vi "InitializeSteering.vi"(8 "error in (no error)":errorcluster, 10 "Steering PID Gains":T1={"proportional gain (Kc)"=100.0, "integral time (Ti, min)"=0.0, "derivative time (Td, min)"=37.0}, 11 "Encoder Initial Position":dbl) -> (0 "error out":errorcluster)   [LabVIEW 2014]
uses:
  <vilib>/Rock Robotics/WPI/CAN/TalonSRX/WPI_CANTalonSRX_APIControlMode.ctl
  <vilib>/Rock Robotics/WPI/CAN/TalonSRX/WPI_CANTalonSRX_APIFeedbackSelect.ctl
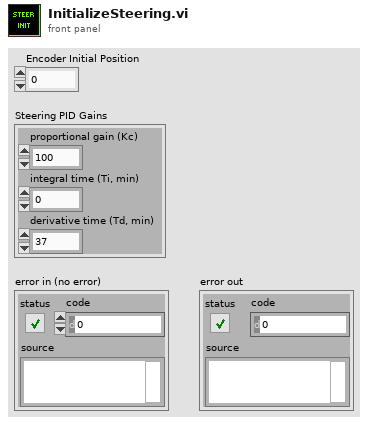
[diagram p1: front panel]
types:
  T1 = cluster{"proportional gain (Kc)":dbl, "integral time (Ti, min)":dbl, "derivative time (Td, min)":dbl}
  T2 = typedef "WPI_CANTalonSRX_APIFeedbackSelect.ctl" = enum16{"Digital Quadrature Encoder", "Analog Potentiometer", "Analog Encoder"}
  T3 = typedef "WPI_CANTalonSRX_APIControlMode.ctl" = enum8{"Percent VBus", "Speed", "Position", "Slave", "Unchanged / Invalid"}
  T4 = typedef "WPI_SwitchDevRef.ctl" = cluster{"DevStatus":errorcluster, "DIO Channel":T5, "Controller":T6, "CntIndex":T7, "Normally Closed":bool}
  T5 = typedef "FPGA_DIOChannel.ctl" = enum8{"DIO 0", "DIO 1", "DIO 2", "DIO 3", "DIO 4", "DIO 5", "DIO 6", "DIO 7", "DIO 8", "DIO 9", "DIO MXP 0", "DIO MXP 1", "DIO MXP 2", "DIO MXP 3", "DIO MXP 4", "DIO MXP 5", "DIO MXP 6", "DIO MXP 7", "DIO MXP 8", "DIO MXP 9", "DIO MXP 10", "DIO MXP 11", "DIO MXP 12", "DIO MXP 13", "DIO MXP 14", "DIO MXP 15", "Invalid"}
  T6 = typedef "FPGA_TypedefDigitalModule.ctl" = enum16{"Controller 1"}
  T7 = typedef "FPGA_CounterCtrSystemIndex.ctl" = enum8{"Ctr 0", "Ctr 1", "Ctr 2", "Ctr 3", "Ctr 4", "Ctr 5", "Ctr 6", "Ctr 7", "Invalid"}
  T8 = typedef "WPI_MotorControlDeviceRef.ctl" = cluster{"DeviceStatus":errorcluster, "Type":T9, "PWM":cluster{"Controller":T6, "PWM Channel":T10, "DeadBand":T11}, "CAN":cluster{"Device Number":u8, "Control Mode":T12, "Semaphore":T13, "Max Vout":dbl, "TalonSRX Control Mode":T3}, "Invert":bool, "TransformRef":T14, "InvTransformRef":T14}
  T9 = typedef "WPI_MotorControlType.ctl" = enum16{"PWM", "CAN", "CANTalonSRX"}
  T10 = typedef "FPGA_DIOPWMChannel.ctl" = enum8{"PWM 0", "PWM 1", "PWM 2", "PWM 3", "PWM 4", "PWM 5", "PWM 6", "PWM 7", "PWM 8", "PWM 9", "PWM MXP 0", "PWM MXP 1", "PWM MXP 2", "PWM MXP 3", "PWM MXP 4", "PWM MXP 5", "PWM MXP 6", "PWM MXP 7", "PWM MXP 8", "PWM MXP 9", "Invalid"}
  T11 = typedef "WPI_PWMDeadband.ctl" = cluster{"Name":string, "maxPositivePwm":i32, "minPositivePwm":i32, "centerPwm":i32, "maxNegativePwm":i32, "minNegativePwm":i32, "angularRange":u16}
  T12 = typedef "WPI_CANJaguar_ControlMode.ctl" = enum8{"Percent VBus", "Current", "Speed", "Position", "Voltage"}
  T13 = typedef "Semaphore RefNum" = refnum<k1>
  T14 = typedef "WPI_PWMTransform_ConPane.ctl" = refnum<vi>
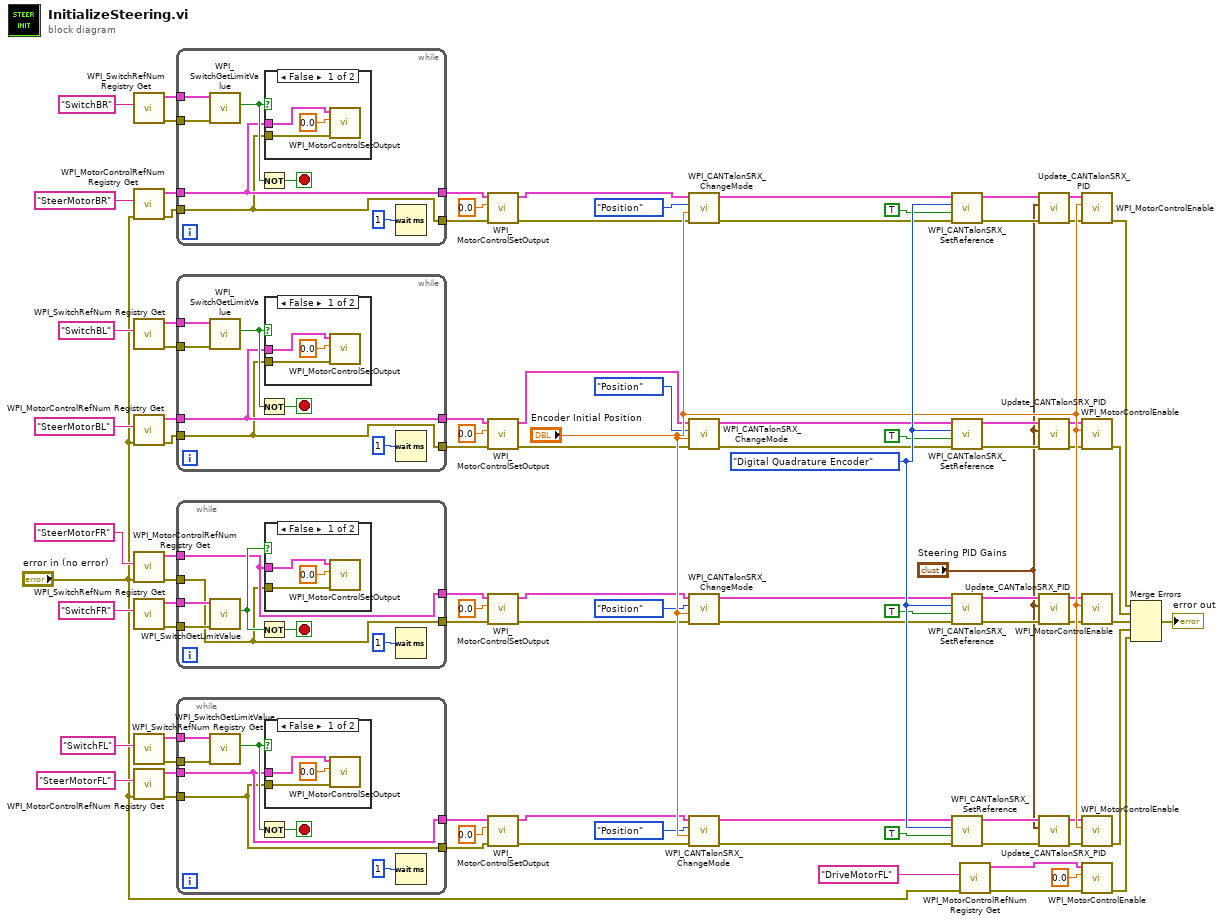
[diagram p0: block diagram]
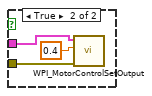
[diagram p2: hidden frame]
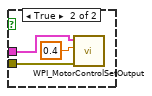
[diagram p3: hidden frame]
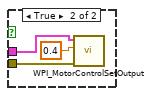
[diagram p4: hidden frame]
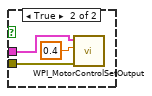
[diagram p5: hidden frame]
diagram:
  w90 = WPI_CANTalonSRX_APIFeedbackSelect."Digital Quadrature Encoder" ("Feedback Reference")
  n1 = call <vilib>:"WPI_SwitchRefNum Registry Get.vi"("refnum name"="SwitchBR") -> ("error out"=w29:errorcluster, "SwitchDevRef"=w28:T4)  [unwired: 9 in]
  n2 = call <vilib>:"WPI_MotorControlRefNum Registry Get.vi"("error in (no error)"="error in (no error)", "refnum name"="SteerMotorBR") -> ("error out"=w13:errorcluster, "MotorControlDevRef"=w14:T8)  [unwired: 8 in]
  n3 = call <vilib>:"WPI_SwitchRefNum Registry Get.vi"("refnum name"="SwitchBL") -> ("error out"=w35:errorcluster, "SwitchDevRef"=w34:T4)  [unwired: 9 in]
  n4 = call <vilib>:"WPI_MotorControlRefNum Registry Get.vi"("error in (no error)"="error in (no error)", "refnum name"="SteerMotorBL") -> ("error out"=w11:errorcluster, "MotorControlDevRef"=w12:T8)  [unwired: 8 in]
  n5 = call <vilib>:"WPI_MotorControlRefNum Registry Get.vi"("error in (no error)"="error in (no error)", "refnum name"="SteerMotorFR") -> ("error out"=w9:errorcluster, "MotorControlDevRef"=w10:T8)  [unwired: 8 in]
  n6 = call <vilib>:"WPI_SwitchRefNum Registry Get.vi"("refnum name"="SwitchFR") -> ("error out"=w17:errorcluster, "SwitchDevRef"=w16:T4)  [unwired: 9 in]
  n7 = call <vilib>:"WPI_SwitchRefNum Registry Get.vi"("refnum name"="SwitchFL") -> ("error out"=w23:errorcluster, "SwitchDevRef"=w22:T4)  [unwired: 9 in]
  n8 = call <vilib>:"WPI_MotorControlRefNum Registry Get.vi"("error in (no error)"="error in (no error)", "refnum name"="SteerMotorFL") -> ("error out"=w7:errorcluster, "MotorControlDevRef"=w8:T8)  [unwired: 8 in]
  n9 = while {
    tunnel: w28 -> [w97]
    tunnel: w29 -> [w96]
    tunnel: w14 -> [w92]
    tunnel: [w92] -> w32
    tunnel: w13 -> [w91]
    tunnel: [w91] -> w30
    stop <- w95 stop-if-true
    n10 = call <vilib>:"WPI_SwitchGetLimitValue.vi"("error in (no error)"=w96, "SwitchDevRef"=w97) -> ("Switch Pressed"=w93:bool)  [unwired: 7 in, 2 out]
    n11 = Not(x=w93) -> (.not. x?=w95:bool)
    n12 = case shown="False" w93 {
      tunnel: w92 -> [w99 w102]
      tunnel: w91 -> [w98 w101]
      frame False {
        n13 = call <vilib>:"WPI_MotorControlSetOutput.vi"("error in (no error)"=w98, "Output"=0.0, "MotorControlDevRef"=w99) -> ()  [unwired: 6 in, 3 out]
      }
      frame True {
        n14 = call <vilib>:"WPI_MotorControlSetOutput.vi"("error in (no error)"=w101, "Output"=0.4, "MotorControlDevRef"=w102) -> ()  [unwired: 6 in, 3 out]
      }
    }
    n15 = Wait (ms)(milliseconds to wait=u32 1) -> ()  [unwired: 1 out]
  }
  n16 = while {
    tunnel: w34 -> [w110]
    tunnel: w35 -> [w109]
    tunnel: w12 -> [w105]
    tunnel: [w105] -> w38
    tunnel: w11 -> [w104]
    tunnel: [w104] -> w36
    stop <- w108 stop-if-true
    n17 = call <vilib>:"WPI_SwitchGetLimitValue.vi"("error in (no error)"=w109, "SwitchDevRef"=w110) -> ("Switch Pressed"=w106:bool)  [unwired: 7 in, 2 out]
    n18 = Not(x=w106) -> (.not. x?=w108:bool)
    n19 = case shown="False" w106 {
      tunnel: w105 -> [w112 w115]
      tunnel: w104 -> [w111 w114]
      frame False {
        n20 = call <vilib>:"WPI_MotorControlSetOutput.vi"("error in (no error)"=w111, "Output"=0.0, "MotorControlDevRef"=w112) -> ()  [unwired: 6 in, 3 out]
      }
      frame True {
        n21 = call <vilib>:"WPI_MotorControlSetOutput.vi"("error in (no error)"=w114, "Output"=0.4, "MotorControlDevRef"=w115) -> ()  [unwired: 6 in, 3 out]
      }
    }
    n22 = Wait (ms)(milliseconds to wait=u32 1) -> ()  [unwired: 1 out]
  }
  n23 = while {
    tunnel: w16 -> [w123]
    tunnel: w17 -> [w122]
    tunnel: w10 -> [w118]
    tunnel: [w118] -> w20
    tunnel: w9 -> [w117]
    tunnel: [w117] -> w18
    stop <- w121 stop-if-true
    n24 = call <vilib>:"WPI_SwitchGetLimitValue.vi"("error in (no error)"=w122, "SwitchDevRef"=w123) -> ("Switch Pressed"=w119:bool)  [unwired: 7 in, 2 out]
    n25 = Not(x=w119) -> (.not. x?=w121:bool)
    n26 = case shown="False" w119 {
      tunnel: w118 -> [w125 w128]
      tunnel: w117 -> [w124 w127]
      frame False {
        n27 = call <vilib>:"WPI_MotorControlSetOutput.vi"("error in (no error)"=w124, "Output"=0.0, "MotorControlDevRef"=w125) -> ()  [unwired: 6 in, 3 out]
      }
      frame True {
        n28 = call <vilib>:"WPI_MotorControlSetOutput.vi"("error in (no error)"=w127, "Output"=0.4, "MotorControlDevRef"=w128) -> ()  [unwired: 6 in, 3 out]
      }
    }
    n29 = Wait (ms)(milliseconds to wait=u32 1) -> ()  [unwired: 1 out]
  }
  n30 = while {
    tunnel: w22 -> [w136]
    tunnel: w23 -> [w135]
    tunnel: w8 -> [w131]
    tunnel: [w131] -> w26
    tunnel: w7 -> [w130]
    tunnel: [w130] -> w24
    stop <- w134 stop-if-true
    n31 = call <vilib>:"WPI_SwitchGetLimitValue.vi"("error in (no error)"=w135, "SwitchDevRef"=w136) -> ("Switch Pressed"=w132:bool)  [unwired: 7 in, 2 out]
    n32 = Not(x=w132) -> (.not. x?=w134:bool)
    n33 = case shown="False" w132 {
      tunnel: w131 -> [w138 w141]
      tunnel: w130 -> [w137 w140]
      frame False {
        n34 = call <vilib>:"WPI_MotorControlSetOutput.vi"("error in (no error)"=w137, "Output"=0.0, "MotorControlDevRef"=w138) -> ()  [unwired: 6 in, 3 out]
      }
      frame True {
        n35 = call <vilib>:"WPI_MotorControlSetOutput.vi"("error in (no error)"=w140, "Output"=0.4, "MotorControlDevRef"=w141) -> ()  [unwired: 6 in, 3 out]
      }
    }
    n36 = Wait (ms)(milliseconds to wait=u32 1) -> ()  [unwired: 1 out]
  }
  n37 = call <vilib>:"WPI_MotorControlSetOutput.vi"("error in (no error)"=w30, "Output"=0.0, "MotorControlDevRef"=w32) -> ("error out"=w44:errorcluster, "MotorControlDevRef"=w45:T8)  [unwired: 6 in, 1 out]
  n38 = call <vilib>:"WPI_MotorControlSetOutput.vi"("error in (no error)"=w36, "Output"=0.0, "MotorControlDevRef"=w38) -> ("error out"=w48:errorcluster, "MotorControlDevRef"=w47:T8)  [unwired: 6 in, 1 out]
  n39 = call <vilib>:"WPI_MotorControlSetOutput.vi"("error in (no error)"=w18, "Output"=0.0, "MotorControlDevRef"=w20) -> ("error out"=w51:errorcluster, "MotorControlDevRef"=w50:T8)  [unwired: 6 in, 1 out]
  n40 = call <vilib>:"WPI_MotorControlSetOutput.vi"("error in (no error)"=w24, "Output"=0.0, "MotorControlDevRef"=w26) -> ("error out"=w54:errorcluster, "MotorControlDevRef"=w53:T8)  [unwired: 6 in, 1 out]
  n41 = call <vilib>:"WPI_CANTalonSRX_ChangeMode.vi"("error in (no error)"=w44, "Output"="Encoder Initial Position", "Control Mode"=WPI_CANTalonSRX_APIControlMode."Position", "CAN Talon SRX Ref"=w45) -> ("error out"=w82:errorcluster, "CAN Talon SRX Ref Out"=w81:T8)  [unwired: 6 in]
  n42 = call <vilib>:"WPI_CANTalonSRX_ChangeMode.vi"("error in (no error)"=w48, "Output"="Encoder Initial Position", "Control Mode"=WPI_CANTalonSRX_APIControlMode."Position", "CAN Talon SRX Ref"=w47) -> ("error out"=w77:errorcluster, "CAN Talon SRX Ref Out"=w76:T8)  [unwired: 6 in]
  n43 = call <vilib>:"WPI_CANTalonSRX_ChangeMode.vi"("error in (no error)"=w51, "Output"="Encoder Initial Position", "Control Mode"=WPI_CANTalonSRX_APIControlMode."Position", "CAN Talon SRX Ref"=w50) -> ("error out"=w70:errorcluster, "CAN Talon SRX Ref Out"=w69:T8)  [unwired: 6 in]
  n44 = call <vilib>:"WPI_CANTalonSRX_ChangeMode.vi"("error in (no error)"=w54, "Output"="Encoder Initial Position", "Control Mode"=WPI_CANTalonSRX_APIControlMode."Position", "CAN Talon SRX Ref"=w53) -> ("error out"=w64:errorcluster, "CAN Talon SRX Ref Out"=w65:T8)  [unwired: 6 in]
  n45 = call <vilib>:"WPI_CANTalonSRX_SetReference.vi"("error in (no error)"=w82, "Reverse Feedback Sensor"=TRUE, "Feedback Reference"=w90, "CAN Talon SRX Ref"=w81) -> ("error out"=w80:errorcluster, "CAN Talon SRX Ref Out"=w79:T8)  [unwired: 6 in]
  n46 = call <vilib>:"WPI_CANTalonSRX_SetReference.vi"("error in (no error)"=w77, "Reverse Feedback Sensor"=TRUE, "Feedback Reference"=w90, "CAN Talon SRX Ref"=w76) -> ("error out"=w75:errorcluster, "CAN Talon SRX Ref Out"=w74:T8)  [unwired: 6 in]
  n47 = call <vilib>:"WPI_CANTalonSRX_SetReference.vi"("error in (no error)"=w70, "Reverse Feedback Sensor"=TRUE, "Feedback Reference"=w90, "CAN Talon SRX Ref"=w69) -> ("error out"=w72:errorcluster, "CAN Talon SRX Ref Out"=w71:T8)  [unwired: 6 in]
  n48 = call <vilib>:"WPI_CANTalonSRX_SetReference.vi"("error in (no error)"=w64, "Reverse Feedback Sensor"=TRUE, "Feedback Reference"=w90, "CAN Talon SRX Ref"=w65) -> ("error out"=w67:errorcluster, "CAN Talon SRX Ref Out"=w66:T8)  [unwired: 6 in]
  n49 = call <vilib>:"WPI_MotorControlRefNum Registry Get.vi"("error in (no error)"="error in (no error)", "refnum name"="DriveMotorFL") -> ("error out"=w1:errorcluster, "MotorControlDevRef"=w5:T8)  [unwired: 8 in]
  n50 = call "Update_CANTalonSRX_PID.vi"("error in (no error)"=w80, "PID Gains"="Steering PID Gains", "CAN Talon SRX Ref"=w79) -> ("error out"=w56:errorcluster, "CAN Talon SRX Ref Out"=w55:T8)  [unwired: 7 in]
  n51 = call "Update_CANTalonSRX_PID.vi"("error in (no error)"=w75, "PID Gains"="Steering PID Gains", "CAN Talon SRX Ref"=w74) -> ("error out"=w58:errorcluster, "CAN Talon SRX Ref Out"=w57:T8)  [unwired: 7 in]
  n52 = call "Update_CANTalonSRX_PID.vi"("error in (no error)"=w72, "PID Gains"="Steering PID Gains", "CAN Talon SRX Ref"=w71) -> ("error out"=w60:errorcluster, "CAN Talon SRX Ref Out"=w59:T8)  [unwired: 7 in]
  n53 = call "Update_CANTalonSRX_PID.vi"("error in (no error)"=w67, "PID Gains"="Steering PID Gains", "CAN Talon SRX Ref"=w66) -> ("error out"=w62:errorcluster, "CAN Talon SRX Ref Out"=w61:T8)  [unwired: 7 in]
  n54 = call <vilib>:"WPI_MotorControlEnable.vi"("error in (no error)"=w56, "Encoder Initial Position"="Encoder Initial Position", "CAN Jaguar Ref"=w55) -> ("error out"=w85:errorcluster)  [unwired: 7 in, 1 out]
  n55 = call <vilib>:"WPI_MotorControlEnable.vi"("error in (no error)"=w58, "Encoder Initial Position"="Encoder Initial Position", "CAN Jaguar Ref"=w57) -> ("error out"=w86:errorcluster)  [unwired: 7 in, 1 out]
  n56 = call <vilib>:"WPI_MotorControlEnable.vi"("error in (no error)"=w60, "Encoder Initial Position"="Encoder Initial Position", "CAN Jaguar Ref"=w59) -> ("error out"=w87:errorcluster)  [unwired: 7 in, 1 out]
  n57 = call <vilib>:"WPI_MotorControlEnable.vi"("error in (no error)"=w62, "Encoder Initial Position"="Encoder Initial Position", "CAN Jaguar Ref"=w61) -> ("error out"=w88:errorcluster)  [unwired: 7 in, 1 out]
  n58 = call <vilib>:"WPI_MotorControlEnable.vi"("error in (no error)"=w1, "Encoder Initial Position"=0.0, "CAN Jaguar Ref"=w5) -> ("error out"=w2:errorcluster)  [unwired: 7 in, 1 out]
  n59 = Merge Errors(w85, w86, w87, w88, w2) -> (→"error out":errorcluster)
